vi "Set Inkscape Ratio.vi"(1 "Image Size In":cluster{"Width":dbl, "Height":dbl}) -> (0 "Image Size Out":cluster{"Width":dbl, "Height":dbl})   [LabVIEW 2019]
uses:
  Global Variables.vi
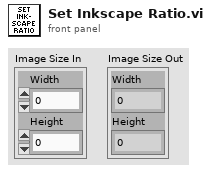
[diagram p1: front panel]
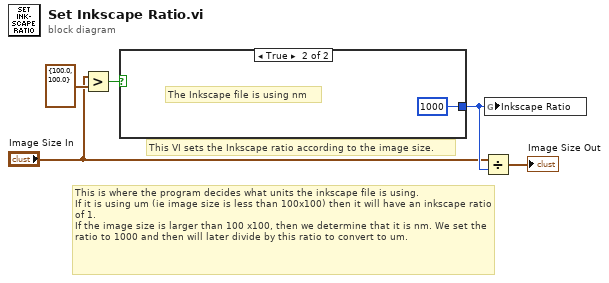
[diagram p0: block diagram]
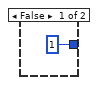
[diagram p2: hidden frame]
diagram:
  # "This is where the program decides what units the inkscape file is using.\nIf it is using um (ie image size is less than 100x100) then it will have an inkscape ratio of 1. \nIf the image size is larger than 100 x100, then we determine that it is nm. We set the ratio to 1000 and then will later divide by this ratio to convert to um."
  # "This VI sets the Inkscape ratio according to the image size."
  n1 = Greater?(x="Image Size In", y=cluster{"Width":dbl, "Height":dbl} {"Width"=100.0, "Height"=100.0}) -> (0:w4:bool)
  n2 = case shown="True" w4 {
    tunnel: [1 1000] -> w3
    frame False {
    }
    frame True {
      # "The Inkscape file is using nm"
    }
  }
  n3 = Divide(x="Image Size In", y=w3) -> (x/y=→"Image Size Out":cluster{"Width":dbl, "Height":dbl})
  n4 = global write "Global Variables.vi" "Inkscape Ratio"(w3) -> ()
